vi "RandomArrayGenerationUsingInitialization.vi"() -> ()   [LabVIEW 2021]
panel:
  in  "Row":i32
  out "2D Array":dbl[][](array[numeric])
  in  "Column":i32
  in  "SIze of the Array":i32
  out "initialized array":dbl[](array[numeric])
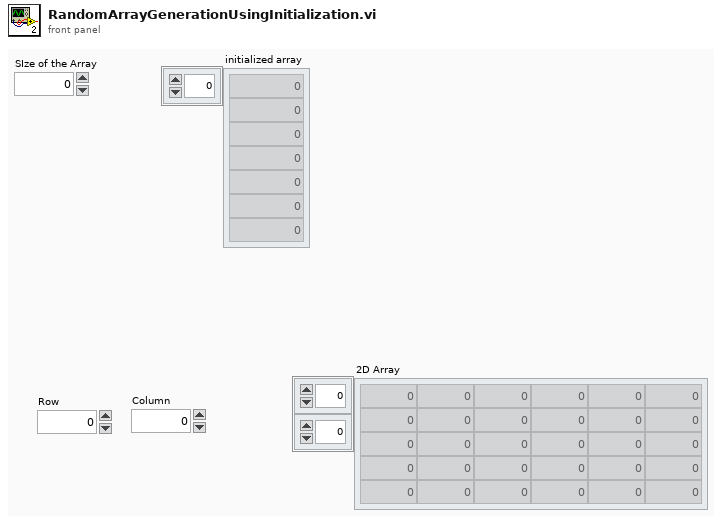
[diagram p1: front panel]
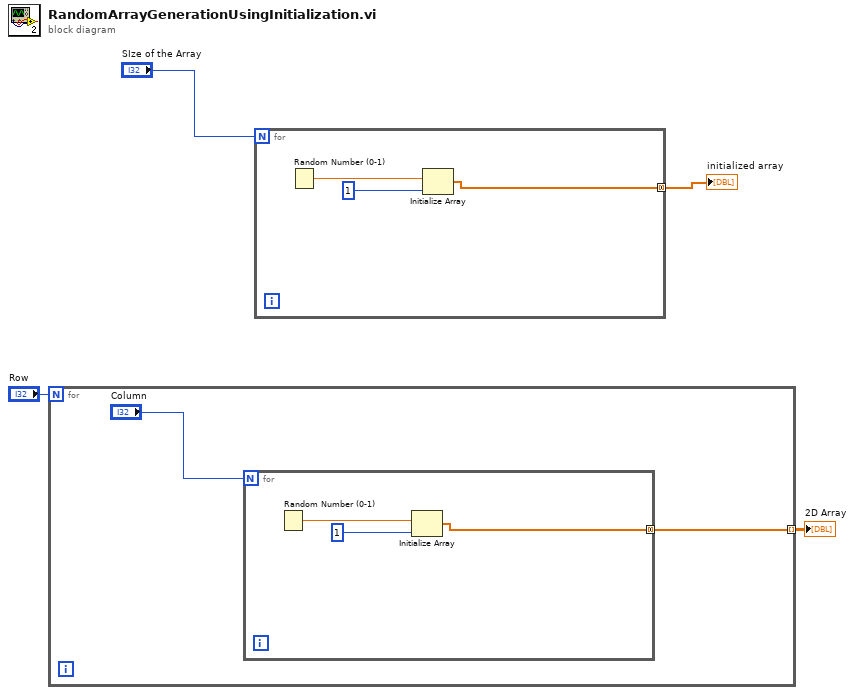
[diagram p0: block diagram]
diagram:
  n1 = for {
    N: "Row" -> [_]
    tunnel: [w5] -> w2 mode=indexing
    n2 = for {
      N: "Column" -> [_]
      tunnel: [w7] -> w5 mode=concatenating
      n3 = Random Number (0-1)() -> (number: 0 to 1=w9:dbl)
      n4 = Initialize Array(w9, 1 ("dimension size")) -> (w7:dbl[])
    }
  }
  "2D Array" <- w2
  n5 = for {
    N: "SIze of the Array" -> [_]
    tunnel: [w10] -> w3 mode=concatenating
    n6 = Random Number (0-1)() -> (number: 0 to 1=w12:dbl)
    n7 = Initialize Array(w12, 1 ("dimension size")) -> (w10:dbl[])
  }
  "initialized array" <- w3
